vi "AVI-Bundle playback parameters.vi"(9 "All header parameters in":T2 {"Pockels" format="%#.6g"; "Software version" format="%#.6g"; "Plane Mode" items=["XY Plane"]; "Angle (degrees)" format="%#.6g"; "Frame Size" items=["100X100"=100, "128X128"=128, "200X200"=200, "256X256"=256, "512X512"=512, "1024x1024"=1024, "2048x2048"=2048]; "Back Apperture" format="%#.6g"; "PMT 2" format="%#.6g"; "PMT 1" format="%#.6g"; "Miniscan Dwell time per pixel (us)" format="%#.6g"; "Zoom" format="%#.6g"; "POI Dwell time (us)" format="%#.6g"; "Acquisition Length (sec)" format="%#.6g"; "Fill time (us)" format="%#.6g"}, 11 "I16 image ref":T1) -> (3 "AVI playback header info cluster":T8)   [LabVIEW 2013]
uses:
  Typedefs/AVI playback header info cluster.ctl
  Functional Imaging Viewer/SubVIs/Experiment header interface/Typedefs/Header parameters cluster-ALL.ctl
  Typedefs/Imaging Protocols enum.ctl
  Typedefs/Frame Size.ctl
  Typedefs/AOL modes.ctl
  Typedefs/Plane Mode.ctl
  Typedefs/Objective selector control enum.ctl
  <vilib>/vision/Image Controls.llb/IMAQ Image.ctl
  Global Variables/General Globals.vi
  <resource>/objmgr/IMAQImage.rc
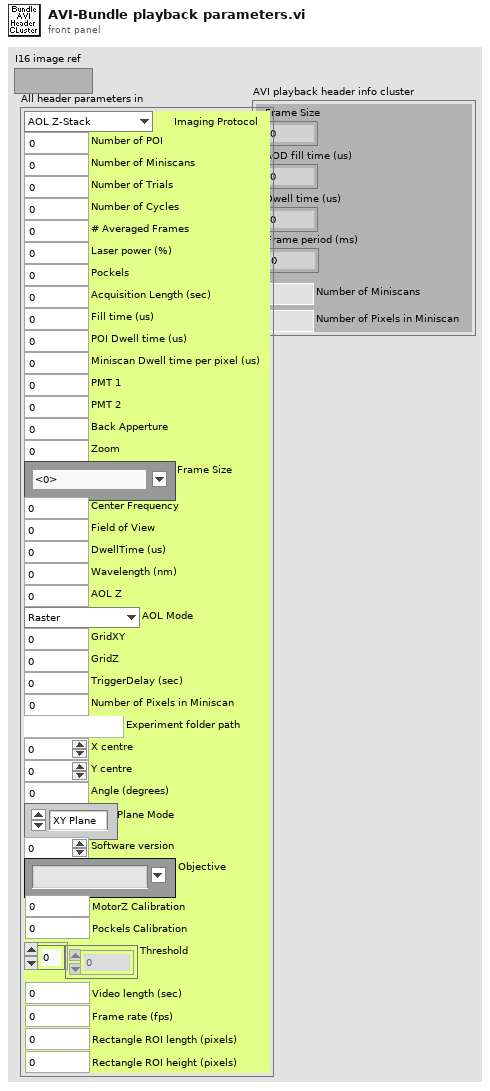
[diagram p1: front panel]
types:
  T1 = typedef "IMAQ Image.ctl" = refnum<image>
  T2 = typedef "Header parameters cluster-ALL.ctl" = cluster{"Imaging Protocol":T3, "Number of POI":u16, "Number of Miniscans":u16, "Number of Trials":u16, "Number of Cycles ":u64, "# Averaged Frames":u16, "Laser power (%)":u8, "Pockels":dbl, "Acquisition Length (sec)":dbl, "Fill time (us)":dbl, "POI Dwell time (us)":dbl, "Miniscan Dwell time per pixel (us)":dbl, "PMT 1":dbl, "PMT 2":dbl, "Back Apperture":dbl, "Zoom":dbl, "Frame Size":T4, "Center Frequency":dbl, "Field of View":dbl, "DwellTime (us)":dbl, "Wavelength (nm)":dbl, "AOL Z":dbl, "AOL Mode":T5, "GridXY":dbl, "GridZ":dbl, "TriggerDelay (sec)":dbl, "Number of Pixels in Miniscan":u16, "Experiment folder path":path, "X centre":dbl, "Y centre":dbl, "Angle (degrees)":dbl, "Plane Mode":T6, "Software version":dbl, "Objective":T7, "MotorZ Calibration":u32, "Pockels Calibration":u32, "Threshold":u16[], "Video length (sec)":dbl, "Frame rate (fps)":u8, "Rectangle ROI length (pixels)":u16, "Rectangle ROI height (pixels)":u16}
  T3 = typedef "Imaging Protocols enum.ctl" = enum16{"AOL Z-Stack", "Motor Z Stack", "Functional Acquisition", "Single Plane Acquisition", "Volume Acquisition", "Live Imaging", "Live Plane Imaging", "Live Volume Imaging"}
  T4 = typedef "Frame Size.ctl" = u16
  T5 = typedef "AOL modes.ctl" = enum16{"Raster", "Structural", "Pointing", "Mini Scan", "Alignment"}
  T6 = typedef "Plane Mode.ctl" = u16
  T7 = typedef "Objective selector control enum.ctl" = string
  T8 = typedef "AVI playback header info cluster.ctl" = cluster{"Frame Size":u32, "AOD fill time (us)":dbl, "Dwell time (us)":dbl, "Frame period (ms)":dbl, "Number of Miniscans":u16, "Number of Pixels in Miniscan":u16}
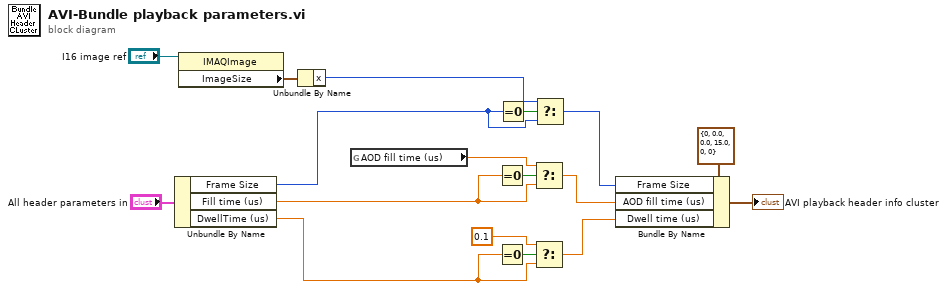
[diagram p0: block diagram]
diagram:
  n1 = Unbundle By Name("All header parameters in") -> ("Frame Size"=w7:T4, "Fill time (us)"=w15:dbl, "DwellTime (us)"=w3:dbl)
  n2 = property class="IMAQImage"(reference="I16 image ref") -> ("ImageSize"=w10:cluster{"x":i32, "y":i32})  [unwired: 1 in, 2 out]
  n3 = Unbundle By Name(w10) -> ("x"=w5:i32)
  n4 = global read "General Globals.vi" "AOD fill time (us)"() -> (w16:dbl)
  n5 = Equal To 0?(x=w15) -> (x = 0?=w13:bool)
  n6 = Equal To 0?(x=w3) -> (x = 0?=w4:bool)
  n7 = Equal To 0?(x=w7) -> (x = 0?=w8:bool)
  n8 = Select(t=w16, s=w13, f=w15) -> (s? t:f=w14:dbl)
  n9 = Select(t=0.1 ("Dwell time (us)"), s=w4, f=w3) -> (s? t:f=w2:dbl)
  n10 = Select(t=w5, s=w8, f=w7) -> (s? t:f=w6:i32)
  n11 = Bundle By Name(cluster=T8 {"Frame Size"=0, "AOD fill time (us)"=0.0, "Dwell time (us)"=0.0, "Frame period (ms)"=15.0, "Number of Miniscans"=0, "Number of Pixels in Miniscan"=0} ("AVI playback header info cluster"), "Frame Size"=w6, "AOD fill time (us)"=w14, "Dwell time (us)"=w2) -> (→"AVI playback header info cluster":T8)
